vi "Initialize RX Transfer.vi"(7 "component name":string, 8 "error in":errorcluster, 9 "timeout (ms)":i32=5000 format="%.0f ms", 11 "Transfer Configuration":refnum<class "Transfer Configuration.lvclass">) -> (0 "error out":errorcluster, 1 "buffer size":i32 format="%d bytes", 2 "timeout?":bool, 3 "transfer parameters":T1)   [LabVIEW 2020, in "RDMA.lvlib" / "RDMA Transceiver.lvclass"]
uses:
  RDMA Transceiver.lvclass
  DSF Core.lvlibp/Classes/Configuration/Core/Transfer/Transfer Configuration.lvclass
  C:/dev/niveristand-data-sharing-framework-custom-device-plugins/Components/DSF Core.lvlibp/Classes/Configuration/Core/Core Configuration.lvclass
  Transfer Parameters.ctl
  Configuration/Rx Transfer/RDMA Transfer Rx Configuration.lvclass
  <vilib>/rdma/rdma.llb/RDMA Direction.ctl
  <vilib>/rdma/rdma.llb/RDMA Configure Buffers U8.vi
  DSF Core.lvlibp/Classes/Configuration/Core/Core Configuration.lvclass
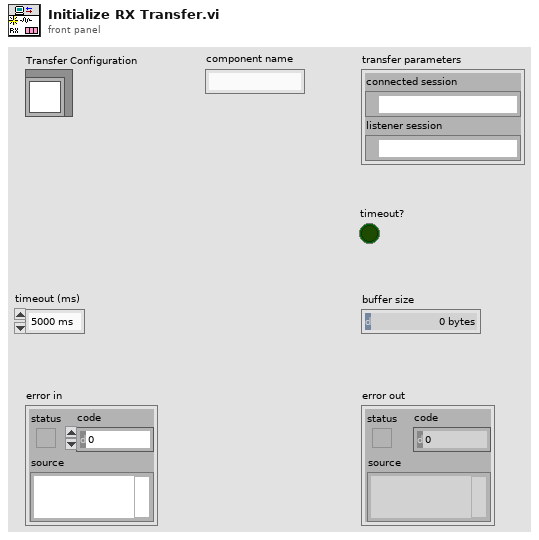
[diagram p1: front panel]
types:
  T1 = typedef "RDMA.lvlib/RDMA Transceiver.lvclass/Transfer Parameters.ctl" = cluster{"connected session":refnum<k21>, "listener session":refnum<k21>}
  T2 = typedef "DSF Core.lvlibp/DSF Settings Info.ctl" = cluster{"component":string, "values":cluster{"key":string, "value":string}[]}
  T3 = typedef "RDMA.lvlib/RDMA Transfer Rx Configuration.lvclass/Rx Transfer Settings.ctl" = cluster{"local address":u32, "local port":u16, "decimation":u16}
  T4 = typedef "RDMA Direction.ctl" = enum16{"Send", "Receive"}
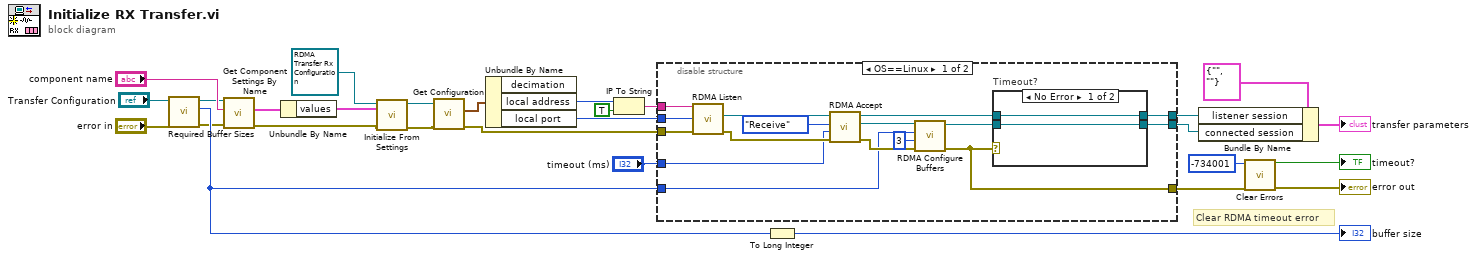
[diagram p0: block diagram]
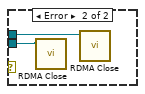
[diagram p2: hidden frame]
diagram:
  # "Clear RDMA timeout error"
  n1 = call-dynamic "Required Buffer Sizes.vi"("error in (no error)"="error in", "Transfer Configuration in"="Transfer Configuration") -> ("error out"=w14:errorcluster, "engine size"=w27:u64, "Transfer Configuration out"=w15:refnum<class "Transfer Configuration.lvclass">)  [unwired: 6 in, 1 out]
  n2 = call "Get Component Settings By Name.vi"("error in (no error)"=w14, "component name"="component name", "Runtime Configuration in"=w15) -> ("error out"=w13:errorcluster, "component settings"=w18:T2)  [unwired: 6 in, 1 out]
  n3 = Unbundle By Name(w18) -> ("values"=w17:cluster{"key":string, "value":string}[])
  n4 = call-dynamic "Initialize From Settings.vi"("error in"=w13, "settings"=w17, "RDMA Rx Transfer Configuration in"=refnum<class "RDMA Transfer Rx Configuration.lvclass"> refnum) -> ("error out"=w22:errorcluster, "RDMA Rx Transfer Configuration out"=w21:refnum<class "RDMA Transfer Rx Configuration.lvclass">)  [unwired: 7 in]
  n5 = call "Get Configuration.vi"("error in"=w22, "RDMA Transfer Rx Configuration in"=w21) -> ("error out"=w12:errorcluster, "transfer settings"=w20:T3)  [unwired: 7 in, 1 out]
  n6 = Unbundle By Name(w20) -> ("local address"=w10:u32, "local port"=w11:u16)  [unwired: 1 out]
  n7 = IP To String(1:TRUE ("dot notation? (F)"), 2:w10) -> (0:w24:string)
  n8 = disable-structure shown="OS==Linux" {
    disable-tunnel: w27 -> [w30 _]
    disable-tunnel: [w32 w49] -> w2
    disable-tunnel: w24 -> [w44 _]
    disable-tunnel: w11 -> [w43 _]
    disable-tunnel: w12 -> [w40 w49]
    disable-tunnel: [w38 _] -> w8
    disable-tunnel: [w33 _] -> w5
    disable-tunnel: "timeout (ms)" -> [w31 _]
    frame condition #0 (active) {
      n9 = call <vilib>:"RDMA Listen.vi"("error in"=w40, "local port"=w43, "local address"=w44) -> ("error out"=w37:errorcluster, "rdma listener session"=w41:refnum<k21>)  [unwired: 6 in, 1 out]
      n10 = call <vilib>:"RDMA Accept.vi"("error in"=w37, "timeout (ms)"=w31, "direction"=RDMA_Direction."Receive", "rdma listener session in"=w41) -> ("error out"=w35:errorcluster, "rdma connected session out"=w36:refnum<k21>, "rdma listener session out"=w39:refnum<k21>)  [unwired: 3 in, 2 out]
      n11 = call-poly <vilib>:"RDMA Configure Buffers.vi"("error in"=w35, "max concurrent transactions"=u64 3, "max transaction size"=w30, "rdma session in"=w36) -> ("error out"=w32:errorcluster, "rdma session out"=w34:refnum<k21>)  [unwired: 6 in]
      n12 = case "Timeout?" shown="No Error" w32 {
        tunnel: w39 -> [w46 w48]
        tunnel: [w46 _] -> w38
        tunnel: w34 -> [w45 w47]
        tunnel: [w45 _] -> w33
        frame No Error {
        }
        frame Error {
          n13 = call <vilib>:"RDMA Close.vi"("rdma session"=w47) -> ()  [unwired: 10 in, 1 out]
          n14 = call <vilib>:"RDMA Close.vi"("rdma session"=w48) -> ()  [unwired: 10 in, 1 out]
        }
      }
    }
    frame condition #1 {
    }
  }
  n15 = To Long Integer(number=w27) -> (32bit integer=→"buffer size":i32)
  n16 = Bundle By Name(cluster=T1 {"connected session"="", "listener session"=""} ("Transfer Tx"), "listener session"=w8, "connected session"=w5) -> (→"transfer parameters":T1)
  n17 = call <vilib>:"Clear Errors.vi"("error in (no error)"=w2, "specific error code to clear (0: all)"=-734001) -> ("error out"=→"error out":errorcluster, "specific error cleared?"=→"timeout?":bool)  [unwired: 4 in]
